vi "Test REQ Socket.vi"(8 "error in (no error)":errorcluster, 11 "RemoteControl.ZMQ in":refnum<class "RemoteControl.ZMQ.lvclass">) -> (0 "error out":errorcluster, 3 "RemoteControl.ZMQ out":refnum<class "RemoteControl.ZMQ.lvclass">)   [LabVIEW 2019, in "RemoteControl.ZMQ.lvclass"]
uses:
  RemoteControl.ZMQ.lvclass
  <vilib>/addons/zeromq/socket_type.ctl
  <vilib>/addons/zeromq/zmq_context.lvclass
  <vilib>/addons/zeromq/zmq_socket.lvclass
  <vilib>/addons/_JKI Toolkits/Caraya/classes/Assert/Assert Not Error.vi
  <vilib>/addons/_JKI Toolkits/Caraya/classes/Assert/Assert Error.vi
  <vilib>/addons/_JKI Toolkits/Caraya/classes/Assert/Assert.lvclass
  <vilib>/addons/zeromq/zeromq.lvlib
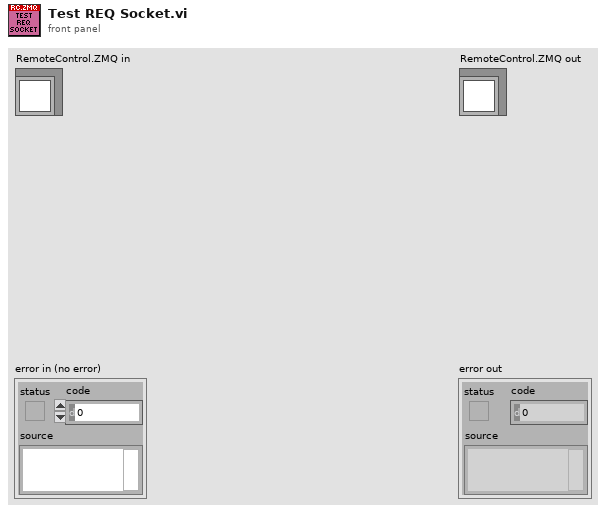
[diagram p1: front panel]
types:
  T1 = typedef "zeromq.lvlib/socket_type.ctl" = enum8{"ZMQ_PAIR", "ZMQ_PUB", "ZMQ_SUB", "ZMQ_REQ", "ZMQ_REP", "ZMQ_DEALER", "ZMQ_ROUTER", "ZMQ_PULL", "ZMQ_PUSH", "ZMQ_XPUB", "ZMQ_XSUB", "ZMQ_STREAM", "ZMQ_SERVER", "ZMQ_CLIENT", "ZMQ_RADIO", "ZMQ_DISH", "ZMQ_GATHER", "ZMQ_SCATTER", "ZMQ_DGRAM"}
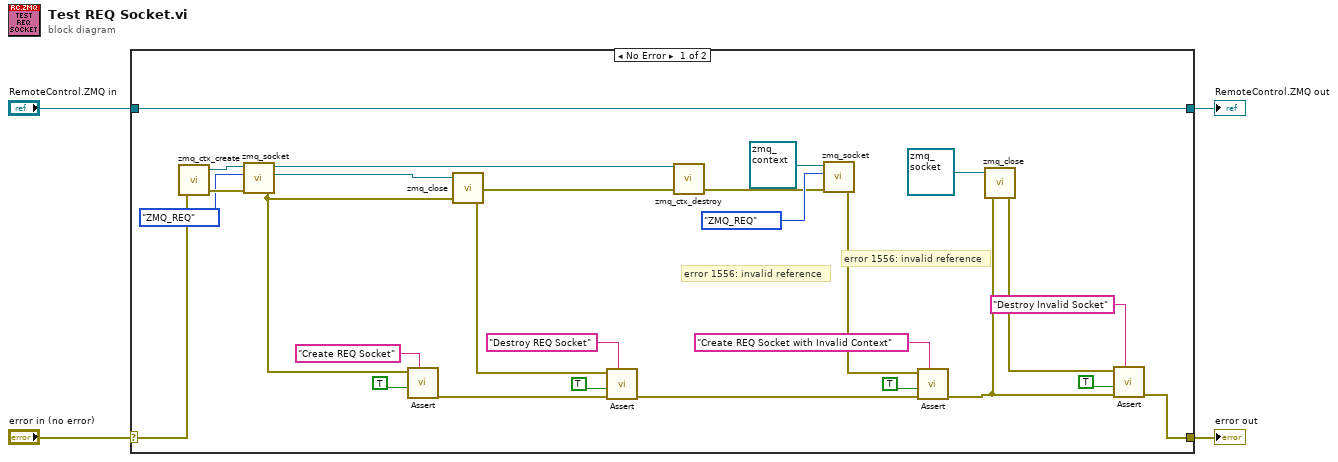
[diagram p0: block diagram]
diagram:
  n1 = case shown="No Error" "error in (no error)" {
    selector: "error in (no error)" -> [w30 w33]
    tunnel: [w5 w33] -> w3
    tunnel: [w24 w32] -> w1
    tunnel: "RemoteControl.ZMQ in" -> [w24 w32]
    frame No Error {
      # "error 1556: invalid reference"
      # "error 1556: invalid reference"
      n2 = call <vilib>:"zmq_ctx_create.vi"("error in"=w30) -> ("error out"=w27:errorcluster, "context out"=w28:refnum<class "zmq_context.lvclass">)  [unwired: 3 in]
      n3 = call <vilib>:"zmq_socket.vi"("error in"=w27, "socket type"=socket_type."ZMQ_REQ", "context in"=w28) -> ("error out"=w19:errorcluster, "socket out"=w25:refnum<class "zmq_socket.lvclass">, "context out"=w23:refnum<class "zmq_context.lvclass">)  [unwired: 2 in]
      n4 = call-poly <vilib>:"Assert.vi"("Label"="Create REQ Socket", "Register with caller test (F)"=TRUE, "Not Error?"=w19) -> ("error out"=w20:errorcluster)  [unwired: 8 in]
      n5 = call <vilib>:"zmq_close.vi"("error in"=w19, "socket"=w25) -> ("error out"=w18:errorcluster)  [unwired: 3 in]
      n6 = call-poly <vilib>:"Assert.vi"("Label"="Destroy REQ Socket", "error in (no error)"=w20, "Register with caller test (F)"=TRUE, "Not Error?"=w18) -> ("error out"=w12:errorcluster)  [unwired: 7 in]
      n7 = call <vilib>:"zmq_ctx_destroy.vi"("error in"=w18, "context in"=w23) -> ("error out"=w15:errorcluster)  [unwired: 3 in]
      n8 = call <vilib>:"zmq_socket.vi"("error in"=w15, "socket type"=socket_type."ZMQ_REQ", "context in"=refnum<class "zmq_context.lvclass"> refnum) -> ("error out"=w11:errorcluster)  [unwired: 2 in, 2 out]
      n9 = call-poly <vilib>:"Assert.vi"("Label"="Create REQ Socket with Invalid Context", "error in (no error)"=w12, "Register with caller test (F)"=TRUE, "Error?"=w11) -> ("error out"=w6:errorcluster)  [unwired: 7 in]
      n10 = call <vilib>:"zmq_close.vi"("error in"=w6, "socket"=refnum<class "zmq_socket.lvclass"> refnum) -> ("error out"=w7:errorcluster)  [unwired: 3 in]
      n11 = call-poly <vilib>:"Assert.vi"("Label"="Destroy Invalid Socket", "error in (no error)"=w6, "Register with caller test (F)"=TRUE, "Error?"=w7) -> ("error out"=w5:errorcluster)  [unwired: 7 in]
    }
    frame Error {
    }
  }
  "error out" <- w3
  "RemoteControl.ZMQ out" <- w1
